vi "Store Panel.vi"(6 "User":string, 8 "error in (no error)":errorcluster, 9 "Show Status? (T)":bool=TRUE, 10 "VI reference":refnum<vi>, 11 "Path (dialog)":path=path "C:/ProgramData/EPL/CFTS Defaults.ini") -> (0 "Error Out":errorcluster)   [LabVIEW 2020]
doc: "Store the values in the controls of a front panel in a file.\n\nFreeware from Moore Good Ideas, www.mooregoodideas.com. Do not remove this line.\ndavid@mooregoodideas.com"
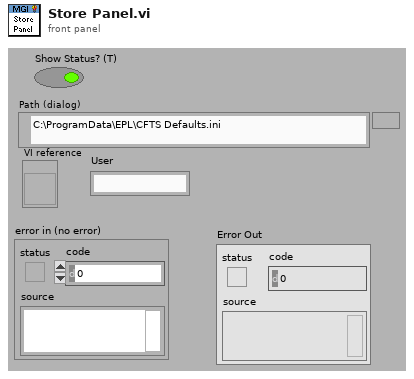
[diagram p1: front panel]
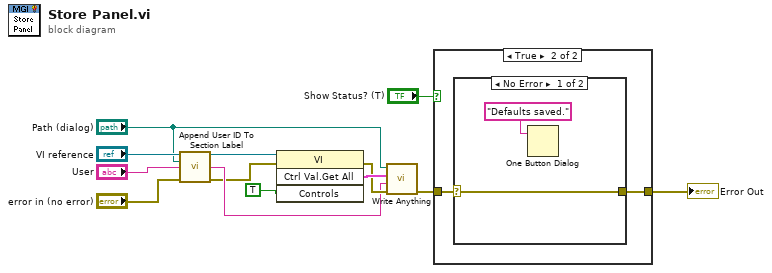
[diagram p0: block diagram]
diagram:
  n1 = call "Append User ID To Section Label.vi"("VI reference"="VI reference", "Path (dialog)"="Path (dialog)", "User"="User", "error in (no error)"="error in (no error)") -> ("VI reference (thru)"=w7:refnum<vi>, "Section Name"=w3:string, "error out"=w2:errorcluster)  [unwired: 8 in, 1 out]
  n2 = invoke class="VI" method="Ctrl Val.Get All"(reference=w7, error in=w2, "Controls"=TRUE) -> (error out=w11:errorcluster, "Get All Control Values Variant"=w13:cluster{"Name":string, "Variant Data":variant}[])  [unwired: 1 in, 2 out]
  n3 = call "Write Anything.vi"("Error In"=w11, "Section Name (Name of \"Anything\")"=w3, "Anything"=w13, "Path (dialog)"="Path (dialog)") -> ("Error Out"=w10:errorcluster)  [unwired: 7 out]
  n4 = case shown="True" "Show Status? (T)" {
    tunnel: w10 -> [w14 w16]
    tunnel: [w14 w15] -> w8
    frame False {
    }
    frame True {
      n5 = case shown="No Error" w16 {
        selector: w16 -> [w17 w19]
        tunnel: [w17 w19] -> w15
        frame No Error {
          n6 = One Button Dialog(message="Defaults saved.") -> ()  [unwired: 1 in, 1 out]
        }
        frame Error {
        }
      }
    }
  }
  "Error Out" <- w8
